vi "HFRR ADV v12.vi"() -> ()   [LabVIEW 2025] (continued)
            n1008 = local write "Temperature On Command"(w1206) -> ()
            n1009 = disable-structure shown="Enabled" {
              disable-tunnel: "Heater On" -> [w1209 _]
              frame Enabled {
                n1010 = local read "EVENT LOG"() -> (w1210:string)
                n1011 = call "Event Log.vi"("Content"=w1209, "EVENT LOG"=w1210) -> ("EVENT LOG"=w1211:string)  [unwired: 8 in, 1 out]
                n1012 = local write "EVENT LOG"(w1211) -> ()
              }
              frame Disabled {
              }
            }
          }
        }
      }
    }
    n1013 = local read "Main Tab"() -> (w936:T2)
    n1014 = case shown="\"About\"" w936 {
      frame "HOME", Default {
        w982 = T16."Enabled" ("Disabled")
        n1015 = local read "Service Password enable"() -> (w981:bool)
        n1016 = property on="Imaging" class="Bool (strict)"("DisabledEnum"=w982) -> ()  [unwired: 2 in, 2 out]
        n1017 = property on="Dashboard" class="Bool (strict)"("DisabledEnum"=w982) -> ()  [unwired: 2 in, 2 out]
        n1018 = property on="Test Setup" class="Bool (strict)"("DisabledEnum"=w982) -> ()  [unwired: 2 in, 2 out]
        n1019 = property on="Analysis" class="Bool (strict)"("DisabledEnum"=w982) -> ()  [unwired: 2 in, 2 out]
        n1020 = property on="Home" class="Bool (strict)"("DisabledEnum"=w982) -> ()  [unwired: 2 in, 2 out]
        n1021 = property on="Report" class="Bool (strict)"("DisabledEnum"=w982) -> ()  [unwired: 2 in, 2 out]
        n1022 = property on="Main Dashboard Buttons" class="RadioBtnsControl (strict)"("DisabledEnum"=w982) -> ()  [unwired: 2 in, 2 out]
        n1023 = case shown="True" w981 {
          tunnel: [T16."Disabled" ("Disabled") T16."Enabled" ("Disabled")] -> w980
          frame False {
          }
          frame True {
          }
        }
        n1024 = property on="About" class="Bool (strict)"("DisabledEnum"=w980) -> ()  [unwired: 2 in, 2 out]
      }
      frame "Test Setup" {
        w987 = T16."Enabled" ("Disabled")
        n1025 = local read "Service Password enable"() -> (w986:bool)
        n1026 = property on="Dashboard" class="Bool (strict)"("DisabledEnum"=T16."Disabled" ("Disabled")) -> ()  [unwired: 2 in, 2 out]
        n1027 = property on="Imaging" class="Bool (strict)"("DisabledEnum"=w987) -> ()  [unwired: 2 in, 2 out]
        n1028 = property on="Analysis" class="Bool (strict)"("DisabledEnum"=w987) -> ()  [unwired: 2 in, 2 out]
        n1029 = property on="Home" class="Bool (strict)"("DisabledEnum"=w987) -> ()  [unwired: 2 in, 2 out]
        n1030 = property on="Report" class="Bool (strict)"("DisabledEnum"=w987) -> ()  [unwired: 2 in, 2 out]
        n1031 = property on="Test Setup" class="Bool (strict)"("DisabledEnum"=w987) -> ()  [unwired: 2 in, 2 out]
        n1032 = case shown="True" w986 {
          tunnel: [T16."Disabled" ("Disabled") T16."Enabled" ("Disabled")] -> w985
          frame False {
          }
          frame True {
          }
        }
        n1033 = property on="About" class="Bool (strict)"("DisabledEnum"=w985) -> ()  [unwired: 2 in, 2 out]
      }
      frame "Adv Scar" {
        w994 = T16."Enabled" ("Disabled")
        n1034 = property on="Dashboard" class="Bool (strict)"("DisabledEnum"=T16."Disabled" ("Disabled")) -> ()  [unwired: 2 in, 2 out]
        n1035 = property on="Imaging" class="Bool (strict)"("DisabledEnum"=w994) -> ()  [unwired: 2 in, 2 out]
        n1036 = property on="Analysis" class="Bool (strict)"("DisabledEnum"=w994) -> ()  [unwired: 2 in, 2 out]
        n1037 = property on="Home" class="Bool (strict)"("DisabledEnum"=w994) -> ()  [unwired: 2 in, 2 out]
        n1038 = property on="Report" class="Bool (strict)"("DisabledEnum"=w994) -> ()  [unwired: 2 in, 2 out]
        n1039 = property on="Test Setup" class="Bool (strict)"("DisabledEnum"=w994) -> ()  [unwired: 2 in, 2 out]
        n1040 = local read "Service Password enable"() -> (w992:bool)
        n1041 = case shown="True" w992 {
          tunnel: [T16."Disabled" ("Disabled") T16."Enabled" ("Disabled")] -> w991
          frame False {
          }
          frame True {
          }
        }
        n1042 = property on="About" class="Bool (strict)"("DisabledEnum"=w991) -> ()  [unwired: 2 in, 2 out]
      }
      frame "Adv Scar Report" {
        w999 = T16."Enabled" ("Disabled")
        n1043 = property on="Dashboard" class="Bool (strict)"("DisabledEnum"=T16."Disabled" ("Disabled")) -> ()  [unwired: 2 in, 2 out]
        n1044 = property on="Imaging" class="Bool (strict)"("DisabledEnum"=w999) -> ()  [unwired: 2 in, 2 out]
        n1045 = property on="Analysis" class="Bool (strict)"("DisabledEnum"=w999) -> ()  [unwired: 2 in, 2 out]
        n1046 = property on="Home" class="Bool (strict)"("DisabledEnum"=w999) -> ()  [unwired: 2 in, 2 out]
        n1047 = property on="Report" class="Bool (strict)"("DisabledEnum"=w999) -> ()  [unwired: 2 in, 2 out]
        n1048 = property on="Test Setup" class="Bool (strict)"("DisabledEnum"=w999) -> ()  [unwired: 2 in, 2 out]
        n1049 = local read "Service Password enable"() -> (w998:bool)
        n1050 = case shown="True" w998 {
          tunnel: [T16."Disabled" ("Disabled") T16."Enabled" ("Disabled")] -> w997
          frame False {
          }
          frame True {
          }
        }
        n1051 = property on="About" class="Bool (strict)"("DisabledEnum"=w997) -> ()  [unwired: 2 in, 2 out]
      }
      frame "Compare Files" {
        w1005 = T16."Enabled" ("Disabled")
        n1052 = local read "Service Password enable"() -> (w1004:bool)
        n1053 = property on="Dashboard" class="Bool (strict)"("DisabledEnum"=T16."Disabled" ("Disabled")) -> ()  [unwired: 2 in, 2 out]
        n1054 = property on="Imaging" class="Bool (strict)"("DisabledEnum"=w1005) -> ()  [unwired: 2 in, 2 out]
        n1055 = property on="Analysis" class="Bool (strict)"("DisabledEnum"=w1005) -> ()  [unwired: 2 in, 2 out]
        n1056 = property on="Home" class="Bool (strict)"("DisabledEnum"=w1005) -> ()  [unwired: 2 in, 2 out]
        n1057 = property on="Report" class="Bool (strict)"("DisabledEnum"=w1005) -> ()  [unwired: 2 in, 2 out]
        n1058 = property on="Test Setup" class="Bool (strict)"("DisabledEnum"=w1005) -> ()  [unwired: 2 in, 2 out]
        n1059 = case shown="True" w1004 {
          tunnel: [T16."Disabled" ("Disabled") T16."Enabled" ("Disabled")] -> w1003
          frame False {
          }
          frame True {
          }
        }
        n1060 = property on="About" class="Bool (strict)"("DisabledEnum"=w1003) -> ()  [unwired: 2 in, 2 out]
      }
      frame "Acquire" {
        n1061 = local read "Service Password enable"() -> (w1009:bool)
        n1062 = property on="Test Setup" class="Bool (strict)"("DisabledEnum"=T16."Disabled" ("Disabled")) -> ()  [unwired: 2 in, 2 out]
        n1063 = local read "Auto Start Test"() -> (w1011:bool)
        n1064 = local read "RUN"() -> (w1013:bool)
        n1065 = case shown="True" w1009 {
          tunnel: [T16."Disabled" ("Disabled") T16."Enabled" ("Disabled")] -> w1010
          frame False {
          }
          frame True {
          }
        }
        n1066 = Or(x=w1013, y=w1011) -> (x .or. y?=w1012:bool)
        n1067 = case shown="True" w1012 {
          tunnel: [T16."Enabled" ("Disabled") T16."Disabled" ("Disabled")] -> w1015
          frame False {
          }
          frame True {
          }
        }
        n1068 = property on="About" class="Bool (strict)"("DisabledEnum"=w1010) -> ()  [unwired: 2 in, 2 out]
        n1069 = property on="Imaging" class="Bool (strict)"("DisabledEnum"=w1015) -> ()  [unwired: 2 in, 2 out]
        n1070 = property on="Dashboard" class="Bool (strict)"("DisabledEnum"=w1015) -> ()  [unwired: 2 in, 2 out]
        n1071 = property on="Analysis" class="Bool (strict)"("DisabledEnum"=w1015) -> ()  [unwired: 2 in, 2 out]
        n1072 = property on="Home" class="Bool (strict)"("DisabledEnum"=w1015) -> ()  [unwired: 2 in, 2 out]
        n1073 = property on="Report" class="Bool (strict)"("DisabledEnum"=w1015) -> ()  [unwired: 2 in, 2 out]
      }
      frame "About" {
        n1074 = local read "FILE"() -> (w1028:string)
        n1075 = local read "TEST FILE NAM,E SAVED"() -> (w1021:bool)
        n1076 = call <vilib>:"Trim Whitespace.vi"("string"=w1028) -> ("trimmed string"=w1027:string)  [unwired: 1 in]
        n1077 = local read "Auto Start Test"() -> (w1031:bool)
        n1078 = String Length(string=w1027) -> (length=w1026:i32)
        n1079 = Greater?(x=w1026, y=1) -> (0:w1023:bool)
        n1080 = And(x=w1023, y=w1021) -> (x .and. y?=w1022:bool)
        n1081 = local read "RUN"() -> (w1033:bool)
        n1082 = case shown="True" w1022 {
          tunnel: [T16."Disabled" ("Disabled") T16."Enabled" ("Disabled")] -> w1024
          frame False {
          }
          frame True {
          }
        }
        n1083 = Or(x=w1033, y=w1031) -> (x .or. y?=w1032:bool)
        n1084 = property on="About" class="Bool (strict)"("DisabledEnum"=T16."Enabled" ("Disabled")) -> ()  [unwired: 2 in, 2 out]
        n1085 = case shown="False" w1032 {
          tunnel: [T16."Enabled" ("Disabled") T16."Disabled" ("Disabled")] -> w1030
          frame False {
          }
          frame True {
          }
        }
        n1086 = property on="Dashboard" class="Bool (strict)"("DisabledEnum"=w1024) -> ()  [unwired: 2 in, 2 out]
        n1087 = property on="Test Setup" class="Bool (strict)"("DisabledEnum"=T16."Disabled" ("Disabled")) -> ()  [unwired: 2 in, 2 out]
        n1088 = property on="Imaging" class="Bool (strict)"("DisabledEnum"=w1030) -> ()  [unwired: 2 in, 2 out]
        n1089 = property on="Analysis" class="Bool (strict)"("DisabledEnum"=w1030) -> ()  [unwired: 2 in, 2 out]
        n1090 = property on="Home" class="Bool (strict)"("DisabledEnum"=w1030) -> ()  [unwired: 2 in, 2 out]
        n1091 = property on="Report" class="Bool (strict)"("DisabledEnum"=w1030) -> ()  [unwired: 2 in, 2 out]
      }
    }
    n1092 = local read "Quit"() -> (w964:bool)
    "Single" <- "Single - Graph"
  }
  n1093 = disable-structure shown="Disabled" {
    disable-tunnel: [w1301 _] -> w36
    disable-tunnel: _ -> [w1300 _]
    frame Disabled {
      n1094 = while {
        tunnel: w1300 -> [_]
        tunnel: [w1302] -> w1301
        tunnel: [w1303] -> _
        i -> [w1303]
        stop <- w1302 stop-if-true
        w1319 = u16 10 items=["1.0"=10, "1.5"=15, "2.0"=20] ("stop bits (10: 1 bit)")
        n1095 = Wait (ms)(milliseconds to wait=u32 10) -> ()  [unwired: 1 out]
        n1096 = call-poly "VISA Configure Serial Port"("VISA resource name"=refnum<visa-resource-name> "ASRL1::INSTR" ("COM PORT"), "timeout (10sec)"=u32 10, "baud rate (9600)"=u32 57600, "data bits (8)"=u16 8, "stop bits (10: 1 bit)"=w1319) -> ("VISA resource name out"=w1305:refnum<visa-resource-name>, "error out"=w1314:errorcluster)  [unwired: 9 in]
        n1097 = VISA Read(VISA resource name=w1305, byte count=u32 2 ("byte count (0)")) -> (read buffer=w1313:string)  [unwired: 1 in, 3 out]
        n1098 = String Subset(string=w1313, offset (0)=0, length (rest)=2 ("length (rest)")) -> (substring=w1312:string)
        n1099 = Match Pattern(string=w1312, regular expression="<>") -> (offset past match=w1309:i32)  [unwired: 1 in, 3 out]
        n1100 = Greater Or Equal?(x=w1309, y=0) -> (x >= y?=w1304:bool)
        n1101 = case shown="True" w1304 {
          tunnel: w1305 -> [_ w1323]
          tunnel: w1314 -> [_ w1322]
          frame False {
          }
          frame True {
            n1102 = VISA Read(VISA resource name=w1323, byte count=u32 32 ("byte count (0)"), error in (no error)=w1322) -> (read buffer=w1321:string)  [unwired: 3 out]
            n1103 = String Subset(string=w1321, offset (0)=0, length (rest)=8 ("length (rest)")) -> (substring=w1325:string)
            n1104 = String Subset(string=w1321, offset (0)=8, length (rest)=8 ("length (rest)")) -> (substring=w1326:string)
            n1105 = Decimal String To Number(string=w1326) -> (number=w1333:i32)  [unwired: 2 in, 1 out]
            n1106 = Decimal String To Number(string=w1325) -> (number=w1329:i32)  [unwired: 2 in, 1 out]
            n1107 = Divide(x=w1333, y=10000) -> ()  [unwired: 1 out]
            n1108 = Divide(x=w1329, y=1000000) -> ()  [unwired: 1 out]
          }
        }
        n1109 = local read "Quit"() -> (w1302:bool)
      }
    }
    frame Enabled {
    }
  }
  n1110 = local write "Err Count"(0 ("Err Count")) -> ()
  n1111 = local write "FRICVALZ"(0.0 ("FRICVALZ")) -> ()
  n1112 = Tick Count (ms)() -> (millisecond timer value=w49:u32)
  n1113 = while {
    shift-right: [w1352] -> w53
    shift-left: _ -> [w1341]
    shift-right: [w1351] -> w52
    shift-left: errorcluster {"status"=TRUE, "code"=0, "source"="Init"} ("error IO") -> [w1343]
    shift-right: [w1349] -> _
    shift-left: w49 -> [w1350]
    tunnel: [w1336] -> w40
    tunnel: [w1348] -> _
    i -> [w1348]
    stop <- w1336 stop-if-true
    n1114 = local read "Com Port 1"() -> (w1342:refnum<visa-resource-name>)
    n1115 = local read "Port 1a"() -> (w1344:bool)
    n1116 = local read "Port 3"() -> (w1345:bool)
    n1117 = Not Equal?(x=w1342, y=w1341) -> (x != y?=w1340:bool)
    n1118 = Or(x=w1345, y=w1344) -> (x .or. y?=w1347:bool)
    n1119 = Unbundle(w1343) -> ("status"=→"Port 3":bool)  [unwired: 2 out]
    n1120 = flat-sequence {
      tunnel: [w1355] -> w1339
      tunnel: w1343 -> [w1355]
      frame #0 {
        n1121 = Wait (ms)(milliseconds to wait=u32 200) -> ()  [unwired: 1 out]
      }
    }
    n1122 = case shown="True" w1347 {
      frame False {
        w1357 = FALSE ("Visible")
        n1123 = property on="Port 1a" class="Bool (strict)"("Visible"=w1357) -> ()  [unwired: 2 in, 2 out]
        n1124 = property on="Port 3" class="Bool (strict)"("Visible"=w1357) -> ()  [unwired: 2 in, 2 out]
      }
      frame True {
        w1358 = TRUE ("Visible")
        n1125 = property on="Port 1a" class="Bool (strict)"("Visible"=w1358) -> ()  [unwired: 2 in, 2 out]
        n1126 = property on="Port 3" class="Bool (strict)"("Visible"=w1358) -> ()  [unwired: 2 in, 2 out]
      }
    }
    n1127 = Or(x=w1340, y="Re-initialize Port1") -> (x .or. y?=w1337:bool)
    n1128 = case shown="True" w1337 {
      tunnel: [w1353 errorcluster {"status"=TRUE, "code"=0, "source"="Init"} ("error out")] -> w1338
      tunnel: w1339 -> [w1353 _]
      frame False {
      }
      frame True {
      }
    }
    n1129 = case shown="No Error" w1338 {
      selector: w1338 -> [w1359 w1704]
      tunnel: [w1364 w1709] -> w1352
      tunnel: [w1363 w1701] -> w1351
      tunnel: w1341 -> [w1362 w1707]
      tunnel: w1350 -> [w1361 w1706]
      tunnel: [w1360 w1706] -> w1349
      frame No Error {
        n1130 = stacked-sequence {
          tunnel: [w1374 _ _ _ _ _] -> w1364
          tunnel: [w1373 _ _ _ _ _] -> w1363
          tunnel: w1362 -> [w1369 _ _ _ _ _]
          tunnel: w1359 -> [w1368 _ _ _ _ _]
          tunnel: w1361 -> [_ w1497 _ _ _ _]
          tunnel: [_ w1496 _ _ _ _] -> w1360
          tunnel: [_ w1468 _ _ _ _] -> _
          frame #0 {
            n1131 = property class="Instr"(reference=w1369, error in=w1368) -> (reference out=w1371:refnum<visa-resource-name>, error out=w1372:errorcluster, "Serial Settings:Number of Bytes at Serial Port"=w1365:u32)
            "Sps 3" <- w1365
            "Port 1" <- w1365
            n1132 = Greater?(x=w1365, y=u32 5) -> (0:w1367:bool)
            n1133 = case shown="True" w1367 {
              tunnel: w1371 -> [w1376 w1403]
              tunnel: w1372 -> [w1375 w1382]
              tunnel: [w1375 w1378] -> w1373
              tunnel: [w1376 w1404] -> w1374
              frame False {
              }
              frame True {
                w1377 = TRUE ("PAUSE")
                w1380 = TRUE ("PAUSE")
                # "Out as Volts"
                n1134 = call "ELAPSED TIMER VI - uno.vi"("error in"=w1382, "RESET"=w1380, "PAUSE"=w1380) -> ("error out"=w1381:errorcluster)  [unwired: 6 in, 2 out]
                n1135 = local read "Residual Uno"() -> (w1397:string)
                n1136 = while {
                  tunnel: [w1452] -> w1379
                  tunnel: [w1451] -> w1404
                  tunnel: w1381 -> [w1450]
                  tunnel: w1403 -> [w1449]
                  tunnel: [w1446] -> _
                  shift-right: [w1442] -> w1385
                  shift-left: w1397 -> [w1444]
                  i -> [w1446]
                  stop <- w1441 stop-if-true
                  w1439 = FALSE ("PAUSE")
                  n1137 = property class="Instr"(reference=w1449, error in=w1450) -> (reference out=w1454:refnum<visa-resource-name>, error out=w1453:errorcluster, "Serial Settings:Number of Bytes at Serial Port"=w1445:u32)
                  n1138 = local read "Quit"() -> (w1440:bool)
                  n1139 = call "ELAPSED TIMER VI - uno.vi"("TARGET"=5.0, "RESET"=w1439, "PAUSE"=w1439) -> ("ELAPSED INDICATION"=w1437:bool)  [unwired: 6 in, 2 out]
                  "ELAPSED INDICATION" <- w1437
                  n1140 = VISA Read(VISA resource name=w1454, byte count=w1445, error in (no error)=w1453) -> (VISA resource name out=w1451:refnum<visa-resource-name>, read buffer=w1443:string, error out=w1452:errorcluster)  [unwired: 1 out]
                  n1141 = Greater?(x=w1445, y=u32 30) -> (0:w1447:bool)
                  n1142 = Concatenate Strings(w1444, w1443) -> (w1442:string)
                  n1143 = Compound Arithmetic op=OR(w1447, w1440, w1437) -> (w1441:bool)
                }
                "UnoRead" <- w1385
                n1144 = call "ELAPSED TIMER VI - uno.vi"("error in"=w1379, "RESET"=w1377, "PAUSE"=w1377) -> ("error out"=w1378:errorcluster)  [unwired: 6 in, 2 out]
                n1145 = while {
                  shift-right: [w1423] -> w1396
                  shift-left: w1385 -> [w1429]
                  tunnel: [w1422] -> w1392 mode=indexing
                  tunnel: [w1424] -> _
                  i -> [w1424]
                  stop <- w1421 stop-if-true
                  n1146 = Match Pattern(string=w1429, regular expression="*") -> (after substring=w1427:string)  [unwired: 1 in, 3 out]
                  n1147 = local read "Quit"() -> (w1420:bool)
                  n1148 = local read "ELAPSED INDICATION"() -> (w1419:bool)
                  n1149 = Match Pattern(string=w1427, regular expression="&") -> (before substring=w1422:string, after substring=w1423:string, offset past match=w1425:i32)  [unwired: 1 in, 1 out]
                  n1150 = Less Than 0?(x=w1425) -> (x < 0?=w1426:bool)
                  n1151 = Compound Arithmetic op=OR(w1426, w1420, w1419) -> (w1421:bool)
                }
                n1152 = local write "Residual Uno"(w1396) -> ()
                n1153 = Array Size(array=w1392) -> (size(s)=w1393:i32)
                n1154 = Decrement(x=w1393) -> (x-1=w1395:i32)
                n1155 = Delete From Array(array=w1392, length=1, index=w1395) -> (array with subset deleted=w1390:string[])  [unwired: 1 out]
                n1156 = Array Size(array=w1390) -> (size(s)=w1389:i32)
                n1157 = Decrement(x=w1389) -> (x-1=w1388:i32)
                n1158 = while {
                  tunnel: [w1418] -> w1401 mode=indexing
                  tunnel: [w1417] -> w1400 mode=indexing
                  tunnel: w1390 -> [w1411] mode=indexing
                  tunnel: w1388 -> [w1410]
                  tunnel: [w1409] -> _
                  i -> [w1409]
                  stop <- w1405 stop-if-true
                  w1412 = 0 ("length (rest)")
                  w1414 = ";" ("regular expression")
                  n1159 = local read "ELAPSED INDICATION"() -> (w1408:bool)
                  n1160 = Less Or Equal?(x=w1410, y=w1409) -> (x <= y?=w1406:bool)
                  n1161 = local read "Quit"() -> (w1407:bool)
                  n1162 = Compound Arithmetic op=OR(w1406, w1407, w1408) -> (w1405:bool)
                  n1163 = Match Pattern(string=w1411, regular expression=w1414) -> (before substring=w1416:string, after substring=w1415:string)  [unwired: 1 in, 2 out]
                  n1164 = Decimal String To Number(string=w1416, default (0L)=w1412) -> (number=w1418:i32)  [unwired: 1 in, 1 out]
                  n1165 = Match Pattern(string=w1415, regular expression=w1414) -> (before substring=w1413:string)  [unwired: 1 in, 3 out]
                  n1166 = Decimal String To Number(string=w1413, default (0L)=w1412) -> (number=w1417:i32)  [unwired: 1 in, 1 out]
                }
                n1167 = case shown="0, Default" "ADC Res" {
                  tunnel: [w1432 w1434] -> w1384
                  frame 0, Default {
                    n1168 = Divide(x=65535 ("length (rest)"), y=2 ("length (rest)")) -> (x/y=w1432:dbl)
                  }
                  frame 1 {
                    n1169 = Divide(x=16777216 ("length (rest)"), y=2 ("length (rest)")) -> (x/y=w1434:dbl)
                  }
                }
                n1170 = Bundle(w1401, w1400) -> (w1391:cluster{i32[], i32[]})  [unwired: 1 in]
                n1171 = Divide(x=w1391, y=w1384) -> (x/y=w1402:cluster{dbl[], dbl[]})
                n1172 = Multiply(x=w1402, y=sgl 5.03 ("Numeric")) -> (x*y=w1399:cluster{dbl[], dbl[]})
                n1173 = Unbundle(w1399) -> (→"Ch1":dbl[], →"Ch0":dbl[])
              }
            }
            n1174 = Not(x=w1367) -> (.not. x?=→"Port 1a":bool)
          }
          frame #1 {
            n1175 = local read "zOff 2"() -> (w1489:dbl)
            n1176 = local read "Ch1"() -> (w1479:dbl[])
            n1177 = case shown="True" "Zero 2" {
              tunnel: w1479 -> [_ w1509]
              frame False {
              }
              frame True {
                n1178 = call-poly <vilib>:"Mean.vi"("X"=w1509) -> ("mean"=→"zOff 2":dbl)  [unwired: 1 out]
                n1179 = local write "Zero 2"(FALSE ("Zero")) -> ()
              }
            }
            n1180 = Subtract(x=w1479, y=w1489) -> (x-y=w1485:dbl[])
            n1181 = call-poly <vilib>:"Mean.vi"("X"=w1479) -> ("mean"=w1480:dbl)  [unwired: 1 out]
            "Slide 3" <- w1480
            n1182 = Multiply(x=w1485, y=1.0 ("PG Oth")) -> (x*y=w1471:dbl[])
            n1183 = local read "FF buffer"() -> (w1476:dbl[])
            n1184 = Divide(x=w1471, y=1) -> (x/y=w1470:dbl[])
            "Fric Val" <- w1470
            n1185 = call <vilib>:"Mean PtByPt.vi"("x"=w1480, "sample length"=10, "initialize"="Reset 2") -> ("mean"=→"Mean Pos Fil 2":dbl)  [unwired: 1 in, 1 out]
            n1186 = Array Size(array=w1476) -> (size(s)=w1478:i32)
            n1187 = call-poly <vilib>:"Mean.vi"("X"=w1470) -> ("mean"=w1484:dbl)  [unwired: 1 out]
            n1188 = Insert Into Array(array=w1476, index=w1478, new element=w1470) -> (w1473:dbl[])
            n1189 = Array Size(array=w1473) -> (size(s)=w1472:i32)
            n1190 = case shown="True" "DC corr 2" {
              tunnel: w1470 -> [w1512 w1515]
              tunnel: [w1512 w1514] -> w1477
              tunnel: w1484 -> [_ w1513]
              frame False {
              }
              frame True {
                n1191 = Subtract(x=w1515, y=w1513) -> (x-y=w1514:dbl[])
              }
            }
            n1192 = Tick Count (ms)() -> (millisecond timer value=w1496:u32)
            n1193 = Greater?(x=w1472, y=1000) -> (0:w1474:bool)
            n1194 = Subtract(x=w1496, y=w1497) -> (x-y=w1495:u32)
            n1195 = case shown="True" w1474 {
              tunnel: [w1502 w1505] -> w1461
              tunnel: w1473 -> [w1502 w1508]
              tunnel: w1472 -> [_ w1507]
              frame False {
              }
              frame True {
                n1196 = Subtract(x=w1507, y=1000) -> (x-y=w1503:i32)
                n1197 = Delete From Array(array=w1508, length=w1503, index=0) -> (array with subset deleted=w1505:dbl[])  [unwired: 1 out]
              }
            }
            n1198 = Divide(x=w1495, y=u32 1000 ("x")) -> (x/y=w1493:dbl)
            n1199 = Array Size(array=w1477) -> (size(s)=w1492:i32)
            n1200 = Divide(x=w1492, y=w1493) -> (x/y=w1488:dbl)
            "Sps 2" <- w1488
            n1201 = Reciprocal(x=w1488) -> (1/x=w1486:dbl)
            "dt" <- w1486
            n1202 = local read "FRIC. FORCE :"() -> (w1458:dbl)
            n1203 = local write "FF buffer"(w1461) -> ()
            n1204 = Negate(x=w1461) -> (-x=w1460:dbl[])
            n1205 = call "Elapsed Time5"("Time Target (s)"="check time s", "Reset"="Reset 3") -> ("Time has Elapsed"=w1463:bool)  [unwired: 10 in, 7 out]
            n1206 = Array Max & Min(array=w1460) -> (max value=w1468:dbl)  [unwired: 3 out]
            n1207 = Bundle By Name("Y"=w1477, "dt"=w1486, "t0"=timestamp(0 s since 1904-01-01)) -> (w1456:waveform(dbl))  [unwired: 1 in]
            n1208 = Multiply(x=w1458, y=21.1986) -> (x*y=w1457:dbl)
            n1209 = Greater Or Equal?(x=w1468, y="Threshold value") -> (x >= y?=w1464:bool)
            n1210 = Multiply(x=w1457, y=w1456) -> (x*y=→"FF_Wfm":waveform(dbl))
            n1211 = And(x=w1464, y=w1463) -> (x .and. y?=w1462:bool)
            n1212 = case shown="True" w1462 {
              frame False {
                n1213 = local write "Reset 3"(FALSE ("Reset 3")) -> ()
              }
              frame True {
                n1214 = local write "Reset 3"(TRUE ("Reset 3")) -> ()
                n1215 = local write "save dpt"(TRUE ("save dpt")) -> ()
              }
            }
          }
          frame #2 {
            n1216 = local read "FF buffer"() -> (w1522:dbl[])
            n1217 = Array Max & Min(array=w1522) -> (max value=w1517:dbl, min value=w1518:dbl)  [unwired: 2 out]
            n1218 = Subtract(x=w1517, y=w1518) -> (x-y=w1519:dbl)
            n1219 = Multiply(x=1.0 ("y 2"), y="Threshold") -> ()  [unwired: 1 out]
            n1220 = Greater?(x=w1519, y="Threshold") -> (0:w1516:bool)
            n1221 = case shown="True" w1516 {
              tunnel: w1522 -> [_ w1529]
              tunnel: [_ w1527] -> _
              frame False {
              }
              frame True {
                w1528 = 1.0 ("y")
                n1222 = Delete From Array(array=w1529, length=100, index=0) -> (deleted portion=w1534:dbl[])  [unwired: 1 out]
                n1223 = call-poly <vilib>:"Mean.vi"("X"=w1534) -> ("mean"=w1533:dbl)  [unwired: 1 out]
                n1224 = Subtract(x=w1529, y=w1533) -> (x-y=w1532:dbl[])
                n1225 = Multiply(x=w1528, y=w1528) -> (x*y=w1530:dbl)
                n1226 = Multiply(x=w1532, y=w1530) -> (x*y=w1531:dbl[])
                "FF cal val" <- w1531
                n1227 = Array Size(array=w1531) -> (size(s)=w1525:i32)
                n1228 = Array Max & Min(array=w1531) -> (max value=w1524:dbl, min value=w1523:dbl)  [unwired: 2 out]
                n1229 = property on="FF Calibration g" class="WFGraph (strict)"("X Scale.Range:Minimum"=0.0 ("y"), "X Scale.Range:Maximum"=w1525, "Y Scale.Range:Minimum"=w1524, "Y Scale.Range:Maximum"=w1523) -> ()  [unwired: 2 in, 2 out]
                n1230 = local read "FRIC. FORCE :"() -> (w1527:dbl)
              }
            }
          }
          frame #3 {
            # "5"
            n1231 = local read "DISPLACEMENT :"() -> (w1625:dbl)
            n1232 = Multiply(x=w1625, y=1.0) -> (x*y=w1543:dbl)
            n1233 = local read "zOff 3"() -> (w1628:dbl)
            n1234 = local read "Ch0"() -> (w1556:dbl[])
            n1235 = case shown="True" "Zero 3" {
              tunnel: w1556 -> [_ w1643]
              frame False {
              }
              frame True {
                n1236 = call-poly <vilib>:"Mean.vi"("X"=w1643) -> ("mean"=→"zOff 3":dbl)  [unwired: 1 out]
                n1237 = local write "Zero 3"(FALSE ("Zero")) -> ()
              }
            }
            n1238 = Add(x=w1556, y="Offset") -> (x+y=w1555:dbl[])
            n1239 = Multiply(x=w1543, y="DISPLACEMENT : 2") -> (x*y=w1610:dbl)
            n1240 = Subtract(x=w1556, y=w1628) -> (x-y=w1613:dbl[])
            n1241 = Multiply(x=w1613, y=w1610) -> (x*y=w1612:dbl[])
            n1242 = Multiply(x=w1613, y=w1543) -> (x*y=w1624:dbl[])
            "ABS DP" <- w1624
            n1243 = local read "Standard Slip Gauge (mm)"() -> (w1611:dbl)
            n1244 = call-poly <vilib>:"Mean.vi"("X"=w1612) -> ("mean"=w1542:dbl)  [unwired: 1 out]
            "Disp (mm)" <- w1542
            "software msrnt" <- w1542
            n1245 = Multiply(x=w1555, y="Gain") -> (x*y=w1550:dbl[])
            "Voltage LVDT Acq" <- w1550
            "gLVDTraw" <- w1550
            n1246 = call-poly <vilib>:"Mean.vi"("X"=w1624) -> ("mean"=w1615:dbl)  [unwired: 1 out]
            n1247 = case shown="True" "DC correction" {
              tunnel: w1624 -> [w1646 w1649]
              tunnel: [w1646 w1648] -> w1562
              tunnel: w1615 -> [_ w1647]
              frame False {
              }
              frame True {
                n1248 = Subtract(x=w1649, y=w1647) -> (x-y=w1648:dbl[])
              }
            }
            n1249 = Divide(x=w1542, y=w1611) -> (x/y=w1609:dbl)
            n1250 = call-poly <vilib>:"Mean.vi"("X"=w1550) -> ("mean"=w1549:dbl)  [unwired: 1 out]
            n1251 = Array Max & Min(array=w1550) -> (max value=w1554:dbl, min value=w1553:dbl)  [unwired: 2 out]
            n1252 = Multiply(x=w1609, y=w1610) -> (x*y=→"DISPLACEMENT : 3":dbl)
            n1253 = Subtract(x=w1554, y=w1553) -> (x-y=→"Pk-Pk":dbl)
            n1254 = local read "dt"() -> (w1627:dbl)
            n1255 = Threshold 1D Array(2:0.0 ("threshold y"), 3:w1562) -> (0:w1579:dbl)  [unwired: 1 in]
            n1256 = Bundle By Name("Y"=w1562, "dt"=w1627, "t0"=timestamp(0 s since 1904-01-01)) -> (w1617:waveform(dbl))  [unwired: 1 in]
            n1257 = local read "FF_Wfm"() -> (w1616:waveform(dbl))
            n1258 = Equal To 0?(x=w1579) -> (x = 0?=w1580:bool)
            n1259 = case shown="True" w1580 {
              tunnel: w1562 -> [_ w1637]
              tunnel: [w1633 w1634] -> w1575
              tunnel: w1579 -> [w1633 _]
              frame False {
              }
              frame True {
                n1260 = Threshold 1D Array(1:20 ("start index (0)"), 2:0.0 ("threshold y"), 3:w1637) -> (0:w1634:dbl)
              }
            }
            n1261 = Build Array(w1617, w1616) -> (w1598:waveform(dbl)[])
            "Waveform Graph 2" <- w1598
            n1262 = call-poly <vilib>:"Extract Single Tone Information.vi"("time signal in"=w1617) -> ("detected amplitude"=w1551:dbl, "detected frequency"=→"RawFreq":dbl)  [unwired: 5 in, 4 out]
            n1263 = Multiply(x=w1551, y=2.0) -> (x*y=w1538:dbl)
            n1264 = Subtract(x=w1549, y="LvdtOff") -> (x-y=w1548:dbl)
            n1265 = local read "StrokeL"() -> (w1539:dbl)
            n1266 = Not A Number/Path/Refnum?(number/path/refnum=w1538) -> (NaN/Path/Refnum?=w1540:bool)
            n1267 = Subtract(x=w1548, y=w1551) -> (x-y=w1560:dbl)
            n1268 = Add(x=w1551, y=w1548) -> (x+y=w1559:dbl)
            n1269 = Index Array(array=w1598) -> (element #1=w1599:waveform(dbl), element #2=w1601:waveform(dbl))  [unwired: 2 in]
            n1270 = Select(t=w1539, s=w1540, f=w1538) -> (s? t:f=w1537:dbl)
            "Stroke" <- w1537
            "Mean(RAW) Stroke" <- w1537
            "StrokeL" <- w1537
            n1271 = Bundle(w1548, w1560, w1559) -> (→"Slide 8":cluster{dbl, dbl, dbl})  [unwired: 1 in]
            n1272 = Unbundle By Name(w1599) -> ("Y"=w1572:dbl[])
            n1273 = Split 1D Array(array=w1562, index=w1575) -> (second subarray=w1576:dbl[])  [unwired: 1 out]
            n1274 = In Range and Coerce(upper limit=1.5, x=w1537, lower limit=0.5) -> (In Range?=w1621:bool)  [unwired: 1 out]
            n1275 = Split 1D Array(array=w1572, index="Window") -> (second subarray=w1590:dbl[])  [unwired: 1 out]
            n1276 = Unbundle By Name(w1601) -> ("Y"=w1573:dbl[])
            n1277 = Threshold 1D Array(1:180 ("start index (0)"), 2:0.0 ("threshold y"), 3:w1576) -> (0:w1574:dbl)
            n1278 = local read "Test \nStatus"() -> (w1618:bool)
            n1279 = Split 1D Array(array=w1573, index=w1575) -> (second subarray=w1570:dbl[])  [unwired: 1 out]
            n1280 = Not(x=w1621) -> (.not. x?=w1620:bool)
            n1281 = call-poly <vilib>:"RMS.vi"("X"=w1590) -> ("rms value"=w1546:dbl)  [unwired: 1 out]
            "Current (A)" <- w1546
            n1282 = Array Max & Min(array=w1590) -> (max value=w1604:dbl, min value=w1605:dbl)  [unwired: 2 out]
            n1283 = Array Max & Min(array=w1573) -> (max value=w1602:dbl, min value=w1603:dbl)  [unwired: 2 out]
            n1284 = Subtract(x=w1604, y=w1605) -> (x-y=w1606:dbl)
            n1285 = Subtract(x=w1602, y=w1603) -> (x-y=w1607:dbl)
            n1286 = And(x=w1620, y=w1618) -> (x .and. y?=w1619:bool)
            n1287 = Split 1D Array(array=w1576, index=w1574) -> (first subarray=w1569:dbl[])  [unwired: 1 out]
            n1288 = Split 1D Array(array=w1570, index=w1574) -> (first subarray=w1567:dbl[])  [unwired: 1 out]
            n1289 = case shown="True" w1619 {
              tunnel: [i32[] [] w1639] -> _
              frame False {
              }
              frame True {
                n1290 = local read "UnoRead"() -> (w1641:string)
                n1291 = local read "Array"() -> (w1642:string[])
                n1292 = Build Array (concatenate)(w1642, w1641) -> (w1640:string[])
                "Array" <- w1640
                n1293 = String Length(string=w1640) -> (length=w1639:i32[])
              }
            }
            n1294 = local read "G_val"() -> (w1592:dbl)
            n1295 = Divide(x=w1607, y=w1606) -> (x/y=w1595:dbl)
            n1296 = call-poly <vilib>:"RMS.vi"("X"=w1567) -> ("rms value"=w1591:dbl)  [unwired: 1 out]
            n1297 = call-poly <vilib>:"Hanning Window.vi"("X"=w1569) -> ("Windowed X"=w1568:dbl[])  [unwired: 1 out]
            n1298 = call-poly <vilib>:"Hanning Window.vi"("X"=w1567) -> ("Windowed X"=w1566:dbl[])  [unwired: 1 out]
            n1299 = local read "Constant (G)"() -> (w1584:dbl)
            n1300 = Divide(x=w1591, y=w1546) -> (x/y=w1585:dbl)
            n1301 = Build Array(w1568, w1566) -> (→"Waveform Graph 4":dbl[][])
            n1302 = Multiply(x=w1595, y=0.2) -> (x*y=w1597:dbl)
            n1303 = Multiply(x=0.8 ("y"), y=w1592) -> (x*y=w1596:dbl)
            n1304 = Add(x=w1597, y=w1596) -> (x+y=w1564:dbl)
            n1305 = Multiply(x=w1585, y=0.2) -> (x*y=w1586:dbl)
            n1306 = Multiply(x=0.8 ("y"), y=w1584) -> (x*y=w1587:dbl)
            n1307 = Add(x=w1586, y=w1587) -> (x+y=w1583:dbl)
            "Constant (G)" <- w1583
            n1308 = Not A Number/Path/Refnum?(number/path/refnum=w1564) -> (NaN/Path/Refnum?=w1563:bool)
            n1309 = Select(t=0.0, s=w1563, f=w1564) -> (s? t:f=w1544:dbl)
            "G_val" <- w1544
            n1310 = Multiply(x=w1546, y=w1544) -> (x*y=→"Friction Force (N)":dbl)
            n1311 = Bundle(w1583, "t"=w1544) -> (→"pk-pk":cluster{dbl, "t":dbl})  [unwired: 1 in]
          }
          frame #4 {
            # "C:\\WinDucom\\data\\"
            # "?C:\\LAB-IQ-NXT\\data"
            n1312 = case shown="True" "save dpt" {
              frame False {
              }
              frame True {
                n1313 = local write "save dpt"(FALSE ("Hold 3")) -> ()
                n1314 = local read "file count"() -> (w1653:i32)
                n1315 = Number To Decimal String(number=w1653) -> (decimal integer string=w1659:string)  [unwired: 1 in]
                n1316 = Add(x=1, y=w1653) -> (x+y=w1654:i32)
                n1317 = local write "file count"(w1654) -> ()
                n1318 = local read "FILE 2"() -> (w1658:string)
                n1319 = Concatenate Strings(w1658, w1659) -> (w1651:string)
                n1320 = Concatenate Strings("C:\\LAB-IQ\\data" ("Substring"), w1651) -> (w1666:string)
                n1321 = local read "FF buffer"() -> (w1661:dbl[])
                n1322 = local read "ABS DP"() -> (w1660:dbl[])
                n1323 = Concatenate Strings(w1666, ".dpf" ("Substring")) -> (w1664:string)
                n1324 = Build Array(w1661, w1660) -> (w1656:dbl[][])
                n1325 = Concatenate Strings("FF ( V ); DP( mincron ) " ("character string"), "\r") -> (w1670:string)
                n1326 = String To Path(string=w1664) -> (path=w1662:path)
                n1327 = Transpose 2D Array(2D array=w1656) -> (transposed array=w1655:dbl[][])
                n1328 = call <vilib>:"Write Characters To File.vi"("append to file? (new file:F)"=FALSE, "character string"=w1670, "file path (dialog if empty)"=w1662) -> ("new file path (Not A Path if cancelled)"=w1667:path)  [unwired: 2 in]
                n1329 = Array To Spreadsheet String(delimiter (Tab)=";", array=w1655, 3:"" ("format string")) -> (spreadsheet string=w1657:string)
                "String 9" <- w1657
                n1330 = call <vilib>:"Write Characters To File.vi"("append to file? (new file:F)"=TRUE, "character string"=w1657, "file path (dialog if empty)"=w1667) -> ()  [unwired: 2 in, 1 out]
              }
            }
          }
          frame #5 {
            n1331 = case shown="True" "Hold 4" {
              frame False {
              }
              frame True {
                n1332 = File Dialog(6:"*.dpf" ("pattern"), 11:path "C:/LAB-IQ" ("start path")) -> (0:w1677:errorcluster, 3:w1692:path)  [unwired: 5 in, 2 out]
                n1333 = Unbundle(w1677) -> ()  [unwired: 3 out]
                n1334 = call <vilib>:"Read Characters From File.vi"("file path (dialog if empty)"=w1692) -> ("character string"=w1682:string)  [unwired: 5 in, 3 out]
                n1335 = Spreadsheet String To Array(delimiter (Tab)=";", format string="%S", spreadsheet string=w1682, array type (2D Dbl)=string[][] []) -> (array=w1686:string[][])
                n1336 = for {
                  tunnel: w1686 -> [w1696] mode=indexing
                  tunnel: [w1695] -> w1687 mode=indexing
                  n1337 = for {
                    tunnel: w1696 -> [w1698] mode=indexing
                    tunnel: [w1697] -> w1695 mode=indexing
                    n1338 = call <vilib>:"Trim Whitespace.vi"("string"=w1698) -> ("trimmed string"=w1697:string)  [unwired: 1 in]
                  }
                }
                n1339 = Fract/Exp String To Number(string=w1687) -> (number=w1689:dbl[][])  [unwired: 3 in, 1 out]
                n1340 = Array Subset(array=w1689, index (row)=1 ("index (col)")) -> (w1691:dbl[][])  [unwired: 3 in]
                n1341 = Index Array(array=w1691, index (col) #1=0 ("disabled index (col)"), index (col) #2=1 ("disabled index (col)")) -> (element #1=w1680:dbl[], element #2=w1679:dbl[])  [unwired: 2 in]
                n1342 = Build Array(w1680, w1679) -> (→"Waveform Graph":dbl[][])
              }
            }
          }
        }
      }
      frame Error {
        w1715 = u16 0 items=["None", "XON/XOFF", "RTS/CTS", "XON/XOFF & RTS/CTS", "DTR/DSR", "XON/XOFF & DTR/DSR"] ("flow control (0:none)  2")
        w1713 = u16 10 items=["1.0"=10, "1.5"=15, "2.0"=20] ("stop bits 2")
        w1711 = u16 0 items=["None", "Odd", "Even", "Mark", "Space"] ("parity 2")
        w1712 = u32 10000  # timeout (10sec)
        n1343 = VISA Close(VISA resource name=w1707, error in (no error)=w1704) -> (error out=w1708:errorcluster)
        n1344 = local write "Sps 3"(0.0 ("Sps 4")) -> ()
        n1345 = local write "Port 1a"(FALSE ("Port 1a")) -> ()
        n1346 = call <vilib>:"Clear Errors.vi"("error in (no error)"=w1708) -> ("error out"=w1705:errorcluster)  [unwired: 5 in, 1 out]
        n1347 = local read "Com Port 1"() -> (w1700:refnum<visa-resource-name>)
        n1348 = call-poly "VISA Configure Serial Port"("VISA resource name"=w1700, "timeout (10sec)"=w1712, "baud rate (9600)"=u32 250000 ("baud rate  2"), "data bits (8)"=u16 8 ("data bits  2"), "parity (0:none)"=w1711, "error in (no error)"=w1705, "stop bits (10: 1 bit)"=w1713, "flow control (0:none)"=w1715) -> ("VISA resource name out"=w1716:refnum<visa-resource-name>, "error out"=w1717:errorcluster)  [unwired: 6 in]
        n1349 = flat-sequence {
          tunnel: w1716 -> [w1719]
          tunnel: w1717 -> [w1718]
          tunnel: [w1719] -> w1709
          tunnel: [w1718] -> w1701
          frame #0 {
            n1350 = Wait (ms)(milliseconds to wait=u32 50) -> ()  [unwired: 1 out]
          }
        }
        "Residual Uno" <- ""
        "Port 1 Error" <- w1701
      }
    }
    n1351 = local read "Quit"() -> (w1336:bool)
    "Error Uno" <- w1343
  }
  n1352 = while {
    shift-right: [w1736] -> w34
    shift-left: _ -> [w1727]
    shift-right: [w1735] -> w33
    shift-left: errorcluster {"status"=FALSE, "code"=0, "source"="Init"} ("error out") -> [w1729]
    tunnel: [w1722] -> w39
    tunnel: [w1734] -> _
    i -> [w1734]
    stop <- w1722 stop-if-true
    n1353 = local read "Com Port 2"() -> (w1728:refnum<visa-resource-name>)
    n1354 = local read "Port 2a"() -> (w1730:bool)
    n1355 = local read "Port 4"() -> (w1731:bool)
    n1356 = Not Equal?(x=w1728, y=w1727) -> (x != y?=w1726:bool)
    n1357 = Or(x=w1731, y=w1730) -> (x .or. y?=w1733:bool)
    n1358 = Unbundle(w1729) -> ("status"=→"Port 4":bool)  [unwired: 2 out]
    n1359 = flat-sequence {
      tunnel: w1729 -> [w1740]
      tunnel: [w1740] -> w1725
      frame #0 {
        n1360 = Wait (ms)(milliseconds to wait=u32 50) -> ()  [unwired: 1 out]
      }
    }
    n1361 = case shown="True" w1733 {
      frame False {
        w1741 = FALSE ("Visible")
        n1362 = property on="Port 2a" class="Bool (strict)"("Visible"=w1741) -> ()  [unwired: 2 in, 2 out]
        n1363 = property on="Port 4" class="Bool (strict)"("Visible"=w1741) -> ()  [unwired: 2 in, 2 out]
      }
      frame True {
        w1742 = TRUE ("Visible")
        n1364 = property on="Port 2a" class="Bool (strict)"("Visible"=w1742) -> ()  [unwired: 2 in, 2 out]
        n1365 = property on="Port 4" class="Bool (strict)"("Visible"=w1742) -> ()  [unwired: 2 in, 2 out]
      }
    }
    n1366 = Or(x=w1726, y="Re-initialize Port2") -> (x .or. y?=w1723:bool)
    n1367 = case shown="True" w1723 {
      tunnel: [w1737 errorcluster {"status"=TRUE, "code"=0, "source"="Init"} ("error out")] -> w1724
      tunnel: w1725 -> [w1737 _]
      frame False {
      }
      frame True {
      }
    }
    n1368 = case shown="No Error" w1724 {
      selector: w1724 -> [w1743 w1903]
      tunnel: [w1745 w1908] -> w1736
      tunnel: [w1744 w1901] -> w1735
      tunnel: w1727 -> [w1747 w1906]
      tunnel: [w1746 _] -> _
      frame No Error {
        n1369 = stacked-sequence {
          tunnel: w1747 -> [w1771 _]
          tunnel: w1743 -> [w1770 _]
          tunnel: [w1757 _] -> w1746
          tunnel: [w1756 _] -> w1745
          tunnel: [w1755 _] -> w1744
          frame #0 {
            n1370 = property class="Instr"(reference=w1771, error in=w1770) -> (reference out=w1754:refnum<visa-resource-name>, error out=w1769:errorcluster, "Serial Settings:Number of Bytes at Serial Port"=w1750:u32)
            "Port 2" <- w1750
            n1371 = Greater?(x=w1750, y=u32 23) -> (0:w1752:bool)
            n1372 = Not(x=w1752) -> ()  [unwired: 1 out]
            n1373 = case shown="True" w1752 {
              tunnel: w1754 -> [w1786 w1811]
              tunnel: w1769 -> [w1785 w1812]
              tunnel: [w1785 w1814] -> w1765
              tunnel: [w1786 w1813] -> w1766
              frame False {
              }
              frame True {
                # "Out as Volts"
                n1374 = local read "Residual Due"() -> (w1810:string)
                n1375 = while {
                  tunnel: [w1860] -> w1814
                  tunnel: [w1859] -> w1813
                  tunnel: w1812 -> [w1858]
                  tunnel: w1811 -> [w1857]
                  tunnel: [w1854] -> _
                  shift-right: [w1852] -> w1809
                  shift-left: w1810 -> [w1851]
                  i -> [w1854]
                  stop <- w1849 stop-if-true
                  n1376 = property class="Instr"(reference=w1857, error in=w1858) -> (reference out=w1862:refnum<visa-resource-name>, error out=w1861:errorcluster, "Serial Settings:Number of Bytes at Serial Port"=w1853:u32)
                  n1377 = local read "Quit"() -> (w1848:bool)
                  n1378 = VISA Read(VISA resource name=w1862, byte count=w1853, error in (no error)=w1861) -> (VISA resource name out=w1859:refnum<visa-resource-name>, read buffer=w1850:string, error out=w1860:errorcluster)  [unwired: 1 out]
                  n1379 = Greater?(x=w1853, y=u32 8) -> (0:w1855:bool)
                  n1380 = Compound Arithmetic op=OR(w1855, w1848) -> (w1849:bool)
                  n1381 = Concatenate Strings(w1851, w1850) -> (w1852:string)
                }
                n1382 = while {
                  shift-right: [w1841] -> w1793
                  shift-left: w1809 -> [w1846]
                  tunnel: [w1840] -> w1805 mode=indexing
                  tunnel: [w1839] -> _
                  i -> [w1839]
                  stop <- w1838 stop-if-true
                  n1383 = Match Pattern(string=w1846, regular expression="*") -> (after substring=w1844:string)  [unwired: 1 in, 3 out]
                  n1384 = local read "Quit"() -> (w1837:bool)
                  n1385 = Match Pattern(string=w1844, regular expression="&") -> (before substring=w1840:string, after substring=w1841:string, offset past match=w1842:i32)  [unwired: 1 in, 1 out]
                  n1386 = Less Than 0?(x=w1842) -> (x < 0?=w1843:bool)
                  n1387 = Compound Arithmetic op=OR(w1843, w1837) -> (w1838:bool)
                }
                n1388 = Array Size(array=w1805) -> (size(s)=w1808:i32)
                n1389 = local write "Residual Due"(w1793) -> ()
                n1390 = Decrement(x=w1808) -> (x-1=w1806:i32)
                n1391 = Delete From Array(array=w1805, length=1, index=w1806) -> (array with subset deleted=w1804:string[])  [unwired: 1 out]
                n1392 = Array Size(array=w1804) -> (size(s)=w1792:i32)
                n1393 = Decrement(x=w1792) -> (x-1=w1791:i32)
                n1394 = while {
                  tunnel: w1804 -> [w1825] mode=indexing
                  tunnel: w1791 -> [w1824]
                  tunnel: [w1822] -> w1799 mode=indexing
                  tunnel: [w1821] -> w1798 mode=indexing
                  tunnel: [w1820] -> w1797 mode=indexing
                  tunnel: [w1819] -> w1796 mode=indexing
                  tunnel: [w1818] -> w1794 mode=indexing
                  tunnel: [w1817] -> _
                  i -> [w1817]
                  stop <- w1816 stop-if-true
                  w1834 = u32 0 ("length (rest)")
                  w1833 = ";" ("regular expression")
                  n1395 = Less Or Equal?(x=w1824, y=w1817) -> (x <= y?=w1823:bool)
                  n1396 = Match Pattern(string=w1825, regular expression=w1833) -> (before substring=w1826:string, after substring=w1827:string)  [unwired: 1 in, 2 out]
                  n1397 = Match Pattern(string=w1827, regular expression=w1833) -> (before substring=w1830:string, after substring=w1828:string)  [unwired: 1 in, 2 out]
                  n1398 = local read "Quit"() -> (w1815:bool)
                  n1399 = Decimal String To Number(string=w1826, default (0L)=w1834) -> (number=w1822:u32)  [unwired: 1 in, 1 out]
                  n1400 = Decimal String To Number(string=w1830, default (0L)=w1834) -> (number=w1821:u32)  [unwired: 1 in, 1 out]
                  n1401 = Match Pattern(string=w1828, regular expression=w1833) -> (before substring=w1831:string, after substring=w1829:string)  [unwired: 1 in, 2 out]
                  n1402 = Decimal String To Number(string=w1831, default (0L)=w1834) -> (number=w1820:u32)  [unwired: 1 in, 1 out]
                  n1403 = Match Pattern(string=w1829, regular expression=w1833) -> (before substring=w1832:string, after substring=w1836:string)  [unwired: 1 in, 2 out]
                  n1404 = Compound Arithmetic op=OR(w1823, w1815) -> (w1816:bool)
                  n1405 = Decimal String To Number(string=w1832, default (0L)=w1834) -> (number=w1819:u32)  [unwired: 1 in, 1 out]
                  n1406 = Decimal String To Number(string=w1836, default (0L)=u8 0 ("length (rest)")) -> (number=w1818:u8)  [unwired: 1 in, 1 out]
                }
                "Din" <- w1794
                n1407 = Bundle(w1799, w1798, w1797, w1796) -> (w1801:cluster{u32[], u32[], u32[], u32[]})  [unwired: 1 in]
                n1408 = Divide(x=w1801, y=4095 ("length (rest)")) -> (x/y=w1803:cluster{dbl[], dbl[], dbl[], dbl[]})
                n1409 = Multiply(x=w1803, y=sgl 3.32 ("Numeric")) -> (x*y=w1795:cluster{dbl[], dbl[], dbl[], dbl[]})
                n1410 = Unbundle(w1795) -> (→"ECR":dbl[], →"Rtemp":dbl[], →"Air temp":dbl[], →"Ch3 2":dbl[])
              }
            }
            n1411 = call "Elapsed Time10"("Time Target (s)"=2.0, "Reset"=w1752, "Auto Reset"=FALSE) -> ("Time has Elapsed"=→"Port 2a":bool)  [unwired: 9 in, 7 out]
            n1412 = local read "Due Com"() -> (w1758:string[])
            n1413 = Array Size(array=w1758) -> (size(s)=w1757:i32)
            n1414 = Delete From Array(array=w1758, length=1, index=0) -> (deleted portion=w1761:string[], array with subset deleted=w1762:string[])
            n1415 = local write "Due Com"(w1762) -> ()
            n1416 = Index Array(array=w1761, index=0) -> (element=w1759:string)
            n1417 = Not Equal?(x=w1759, y="") -> (x != y?=w1767:bool)
            n1418 = case shown="True" w1767 {
              tunnel: w1766 -> [w1773 w1778]
              tunnel: [w1773 w1782] -> w1756
              tunnel: w1765 -> [w1772 w1777]
              tunnel: [w1772 w1780] -> w1755
              tunnel: w1759 -> [_ w1776]
              tunnel: [_ w1779] -> _
              frame False {
                # "DATA  WRITE LOOP"
              }
              frame True {
                n1419 = Concatenate Strings(w1776, "\r\n") -> (w1775:string)
                n1420 = VISA Write(VISA resource name=w1778, write buffer=w1775, error in (no error)=w1777) -> (VISA resource name out=w1782:refnum<visa-resource-name>, return count=w1779:u32, error out=w1781:errorcluster)
                n1421 = flat-sequence {
                  tunnel: w1781 -> [w1783]
                  tunnel: [w1783] -> w1780
                  frame #0 {
                    n1422 = Wait (ms)(milliseconds to wait=u32 5) -> ()  [unwired: 1 out]
                  }
                }
              }
            }
          }
          frame #1 {
            w1871 = 10 ("y")
            w1876 = 10 ("y")
            n1423 = local read "Rtemp"() -> (w1864:dbl[])
            n1424 = local read "ecr buf"() -> (w1865:dbl[])
            n1425 = for {
              tunnel: w1864 -> [w1888] mode=indexing
              shift-right: [w1889] -> w1872
              shift-left: dbl[] [] ("temp buf 2") -> [w1890]
              n1426 = Build Array (concatenate)(w1890, w1888) -> (w1891:dbl[])
              n1427 = Equal To 0?(x=w1888) -> (x = 0?=w1892:bool)
              n1428 = Select(t=w1890, s=w1892, f=w1891) -> (s? t:f=w1889:dbl[])
            }
            n1429 = local read "ECR"() -> (w1863:dbl[])
            n1430 = Insert Into Array(array=w1863, index=0, new element=w1865) -> (w1869:dbl[])
            n1431 = local read "temp buf"() -> (w1873:dbl[])
            n1432 = Array Size(array=w1869) -> (size(s)=w1870:i32)
            n1433 = Greater?(x=w1870, y=w1871) -> (0:w1868:bool)
            n1434 = case shown="True" w1868 {
              tunnel: w1869 -> [w1881 w1887]
              tunnel: w1870 -> [_ w1885]
              tunnel: w1871 -> [_ w1884]
              tunnel: [w1881 w1882] -> w1866
              frame False {
              }
              frame True {
                n1435 = Subtract(x=w1885, y=w1884) -> (x-y=w1883:i32)
                n1436 = Delete From Array(array=w1887, length=w1883, index=0) -> (array with subset deleted=w1882:dbl[])  [unwired: 1 out]
              }
            }
            "ecr buf" <- w1866
            n1437 = Insert Into Array(array=w1872, index=0, new element=w1873) -> (w1878:dbl[])
            n1438 = Array Size(array=w1878) -> (size(s)=w1877:i32)
            n1439 = Greater?(x=w1877, y=w1876) -> (0:w1879:bool)
            n1440 = case shown="True" w1879 {
              tunnel: w1878 -> [w1893 w1899]
              tunnel: w1877 -> [_ w1897]
              tunnel: w1876 -> [_ w1896]
              tunnel: [w1893 w1894] -> w1875
              frame False {
              }
              frame True {
                n1441 = Subtract(x=w1897, y=w1896) -> (x-y=w1895:i32)
                n1442 = Delete From Array(array=w1899, length=w1895, index=0) -> (array with subset deleted=w1894:dbl[])  [unwired: 1 out]
              }
            }
            "temp buf" <- w1875
          }
        }
      }
      frame Error {
        w1914 = u16 0 items=["None", "XON/XOFF", "RTS/CTS", "XON/XOFF & RTS/CTS", "DTR/DSR", "XON/XOFF & DTR/DSR"] ("flow control (0:none)  2")
        w1912 = u16 10 items=["1.0"=10, "1.5"=15, "2.0"=20] ("stop bits 2")
        w1910 = u16 0 items=["None", "Odd", "Even", "Mark", "Space"] ("parity 2")
        w1911 = u32 10000  # timeout (10sec)
        n1443 = VISA Clear(VISA resource name=w1906, error in (no error)=w1903) -> (VISA resource name out=w1905:refnum<visa-resource-name>, error out=w1904:errorcluster)
        n1444 = VISA Close(VISA resource name=w1905, error in (no error)=w1904) -> (error out=w1907:errorcluster)
        n1445 = call <vilib>:"Clear Errors.vi"("error in (no error)"=w1907) -> ()  [unwired: 5 in, 2 out]
        n1446 = local read "Com Port 2"() -> (w1900:refnum<visa-resource-name>)
        "visa due" <- w1900
        n1447 = call-poly "VISA Configure Serial Port"("VISA resource name"=w1900, "timeout (10sec)"=w1911, "baud rate (9600)"=u32 250000 ("baud rate  2"), "data bits (8)"=u16 8 ("data bits  2"), "parity (0:none)"=w1910, "stop bits (10: 1 bit)"=w1912, "flow control (0:none)"=w1914) -> ("VISA resource name out"=w1915:refnum<visa-resource-name>, "error out"=w1916:errorcluster)  [unwired: 7 in]
        n1448 = flat-sequence {
          tunnel: w1915 -> [w1918]
          tunnel: w1916 -> [w1917]
          tunnel: [w1918] -> w1908
          tunnel: [w1917] -> w1901
          frame #0 {
            n1449 = Wait (ms)(milliseconds to wait=u32 50) -> ()  [unwired: 1 out]
          }
        }
        "Residual Due" <- ""
        "Port 2 Error" <- w1901
      }
    }
    n1450 = local read "Quit"() -> (w1722:bool)
    "Error Due" <- w1729
  }
  n1451 = property on="RUN" class="Bool (strict)"("Visible"=TRUE) -> ()  [unwired: 2 in, 2 out]
  n1452 = while {
    tunnel: [w1936] -> _
    tunnel: [w1920] -> w55
    i -> [w1936]
    stop <- w1920 stop-if-true
    n1453 = local read "conststatus"() -> (w1924:dbl)
    n1454 = local read "Main Tab"() -> (w1922:T2)
    n1455 = local read "EDIT"() -> (w1942:bool)
    n1456 = local read "Rate"() -> (w1941:dbl)
    n1457 = case shown="True" w1942 {
      tunnel: [FALSE TRUE] -> w1928
      frame False {
      }
      frame True {
      }
    }
    n1458 = property on="Time slide" class="Slide (strict)"("Scale.Range:Maximum"=2500.0) -> ()  [unwired: 2 in, 2 out]
    n1459 = Equal?(x=w1922, y=T23."About" ("Main Tab")) -> (x = y?=w1934:bool)
    n1460 = Equal?(x=w1924, y=0.0) -> (x = y?=w1925:bool)
    n1461 = Divide(x=1.0, y=w1941) -> (x/y=w1937:dbl)
    "Time 2" <- w1937
    n1462 = case shown="True" w1925 {
      frame False {
      }
      frame True {
        # "C:\\WinDucom\\calibrate WO 2391.dcf"
        n1463 = local write "Lan flag"(22) -> ()
        n1464 = local write "conststatus"(10.0 ("rpm value : 2")) -> ()
        n1465 = String To Path(string="C:\\LAB-IQ\\calibrate WO 2465.dcf") -> (path=w1948:path)
        n1466 = Open/Create/Replace File "Open File"(file path (use dialog)=w1948) -> (refnum out=w1946:refnum<file>)  [unwired: 5 in, 2 out]
        n1467 = for {
          N: 23 -> [_]
          tunnel: w1946 -> [w1957]
          i -> [w1951]
          (unwired) TRUE ("line mode (F)")
          n1468 = Read from Text File "Read File"(file (use dialog)=w1957) -> (text=w1956:string)  [unwired: 3 in, 3 out]
          n1469 = Match Pattern(string=w1956, regular expression="]") -> (after substring=w1954:string)  [unwired: 1 in, 3 out]
          n1470 = String Subset(string=w1956, offset (0)=5, length (rest)=10 ("length (rest)")) -> (substring=w1949:string)
          n1471 = Fract/Exp String To Number(string=w1949) -> (number=w1950:dbl)  [unwired: 3 in, 1 out]
          n1472 = Match Pattern(string=w1954, regular expression="-") -> (before substring=w1952:string)  [unwired: 1 in, 3 out]
          n1473 = case shown="8" w1951 {
            tunnel: w1950 -> [w1960 w1961 w1962 w1963 _ _ _ w1968 w1969 w1970 w1973 w1974 w1975 w1976 w1977 w1978 w1979 w1982 w1983 _ _ w1986 _ _]
            tunnel: w1952 -> [_ _ _ _ w1964 w1965 w1966 _ _ _ _ _ _ _ _ _ _ _ _ w1984 w1985 _ w1987 _]
            frame 0 {
              n1474 = local write "FRIC. FORCE :"(w1960) -> ()
            }
            frame 1 {
              n1475 = local write "TEMPERATURE :"(w1961) -> ()
            }
            frame 2 {
              n1476 = local write "HUMIDITY:"(w1962) -> ()
            }
            frame 3 {
              n1477 = local write "AIR TEMPERATURE :"(w1963) -> ()
            }
            frame 4 {
              n1478 = local write "Com Port 1"(w1964) -> ()
            }
            frame 5 {
              n1479 = local write "Com Port 2"(w1965) -> ()
              n1480 = local write "visa due"(w1965) -> ()
            }
            frame 6 {
              n1481 = String To Path(string=w1966) -> (path=w1967:path)
              n1482 = local write "File Path"(w1967) -> ()
              "String" <- w1966
            }
            frame 7 {
              n1483 = local write "DISPLACEMENT :"(w1968) -> ()
            }
            frame 8 {
              n1484 = local write "STROKE GAIN :"(w1969) -> ()
            }
            frame 9 {
              n1485 = local read "Stroke PID Gains"() -> (w1972:T9)
              n1486 = Bundle By Name(cluster=w1972, "Proportional Gain (Kc)"=w1970) -> (w1971:T9)
              n1487 = local write "Stroke PID Gains"(w1971) -> ()
            }
            frame 10 {
              n1488 = local write "Language Selection"(w1973) -> ()
            }
            frame 11 {
              n1489 = local write "CH-POWER +"(w1974) -> ()
            }
            frame 12 {
              n1490 = local write "CH-POWER -"(w1975) -> ()
            }
            frame 13 {
              n1491 = local write "CH-HEATER"(w1976) -> ()
            }
            frame 14 {
              n1492 = local write "CH-HUMIDITY WET"(w1977) -> ()
            }
            frame 15 {
              n1493 = local write "CH-HUMIDITY DRY"(w1978) -> ()
            }
            frame 16 {
              n1494 = local read "Stroke PID Gains"() -> (w1981:T9)
              n1495 = Bundle By Name(cluster=w1981, "Integral Time (Ti, min)"=w1979) -> (w1980:T9)
              n1496 = local write "Stroke PID Gains"(w1980) -> ()
            }
            frame 17 {
              n1497 = local write "AIR TEMP INTERCEPT:"(w1982) -> ()
            }
            frame 18 {
              n1498 = local write "TEMP INTERCEPT:"(w1983) -> ()
            }
            frame 19 {
              n1499 = local write "S.NO"(w1984) -> ()
            }
            frame 20 {
              n1500 = local write "Com Port 3"(w1985) -> ()
            }
            frame 21 {
              n1501 = local write "LvdtOff"(w1986) -> ()
            }
            frame 22 {
              n1502 = local write "C3 :"(w1987) -> ()
            }
            frame 23, Default {
            }
          }
        }
      }
    }
    n1503 = Select(t=u32 2500 ("milliseconds to wait"), s=w1934, f=u32 500 ("milliseconds to wait")) -> (s? t:f=w1932:u32)
    n1504 = Multiply(x=w1937, y=w1932) -> (x*y=w1939:dbl)
    n1505 = property on="FF Calibration g" class="WFGraph (strict)"("Visible"=w1928) -> ()  [unwired: 2 in, 2 out]
    n1506 = property on="Lift" class="Bool (strict)"("Visible"=w1928) -> ()  [unwired: 2 in, 2 out]
    n1507 = property on="Threshold" class="DigNum (strict)"("Visible"=w1928) -> ()  [unwired: 2 in, 2 out]
    n1508 = property on="Time slide" class="Slide (strict)"("Visible"=w1928) -> ()  [unwired: 2 in, 2 out]
    n1509 = call "Elapsed Time2"("Time Target (s)"=w1939, "Auto Reset"=TRUE) -> ("Time has Elapsed"=w1929:bool)  [unwired: 10 in, 7 out]
    n1510 = case shown="True" w1929 {
      frame False {
        # "79.77669138"
        # "2.3554"
        n1511 = local read "FRIC. FORCE :"() -> (w1992:dbl)
        n1512 = local read "FF cal val"() -> (w1989:dbl[])
        n1513 = Multiply(x=w1992, y=79.77669138) -> (x*y=w1991:dbl)
        n1514 = Multiply(x=w1989, y=w1991) -> (x*y=→"FF Calibration g":dbl[])
        "Err Count" <- 0 ("y")
      }
      frame True {
        n1515 = stacked-sequence {
          frame #0 {
            n1516 = stacked-sequence {
              frame #0 {
                "Lift" <- TRUE ("Lift")
              }
            }
          }
          frame #1 {
            w2004 = 2500 ("y")
            n1517 = local read "RUN"() -> (w1996:bool)
            n1518 = local read "FF1"() -> (w1999:dbl[])
            n1519 = case shown="False" w1996 {
              frame False {
                n1520 = local write "Frequency"(0.0 ("Frequency")) -> ()
              }
              frame True {
              }
            }
            n1521 = Array Size(array=w1999) -> (size(s)=w1998:i32)
            n1522 = local read "Ch1"() -> (w1995:dbl[])
            "Waveform Chart 2" <- w1995
            n1523 = call-poly <vilib>:"Mean.vi"("X"=w1995) -> ("mean"=→"Raw Mean":dbl)  [unwired: 1 out]
            n1524 = Insert Into Array(array=w1999, index=w1998, new element=w1995) -> (w2001:dbl[])
            n1525 = Array Size(array=w2001) -> (size(s)=w2005:i32)
            n1526 = Subtract(x=w2005, y=w2004) -> (x-y=w2003:i32)
            n1527 = Greater?(x=w2005, y=w2004) -> (0:w2006:bool)
            n1528 = case shown="True" w2006 {
              tunnel: w2003 -> [_ w2010]
              tunnel: [w2008 w2012] -> w1997
              tunnel: w2001 -> [w2008 w2011]
              frame False {
